vi "Position Removing.vi"(11 "System":string) -> ()   [LabVIEW 2023]
uses:
  <vilib>/Utility/file.llb/Read Delimited Spreadsheet (string).vi
  <vilib>/Utility/file.llb/Write Delimited Spreadsheet (string).vi
panel:
  out "Message":string
  in  "Enter":bool
  in  "Rack Number":i32=1 min=1 max=16 step=1
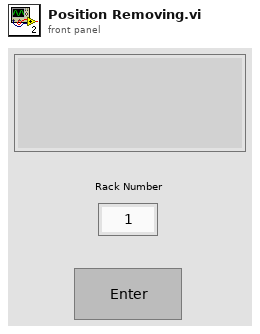
[diagram p1: front panel]
types:
  T1 = enum16{"open", "replace", "create", "open or create", "replace or create", "replace or create with confirmation"}
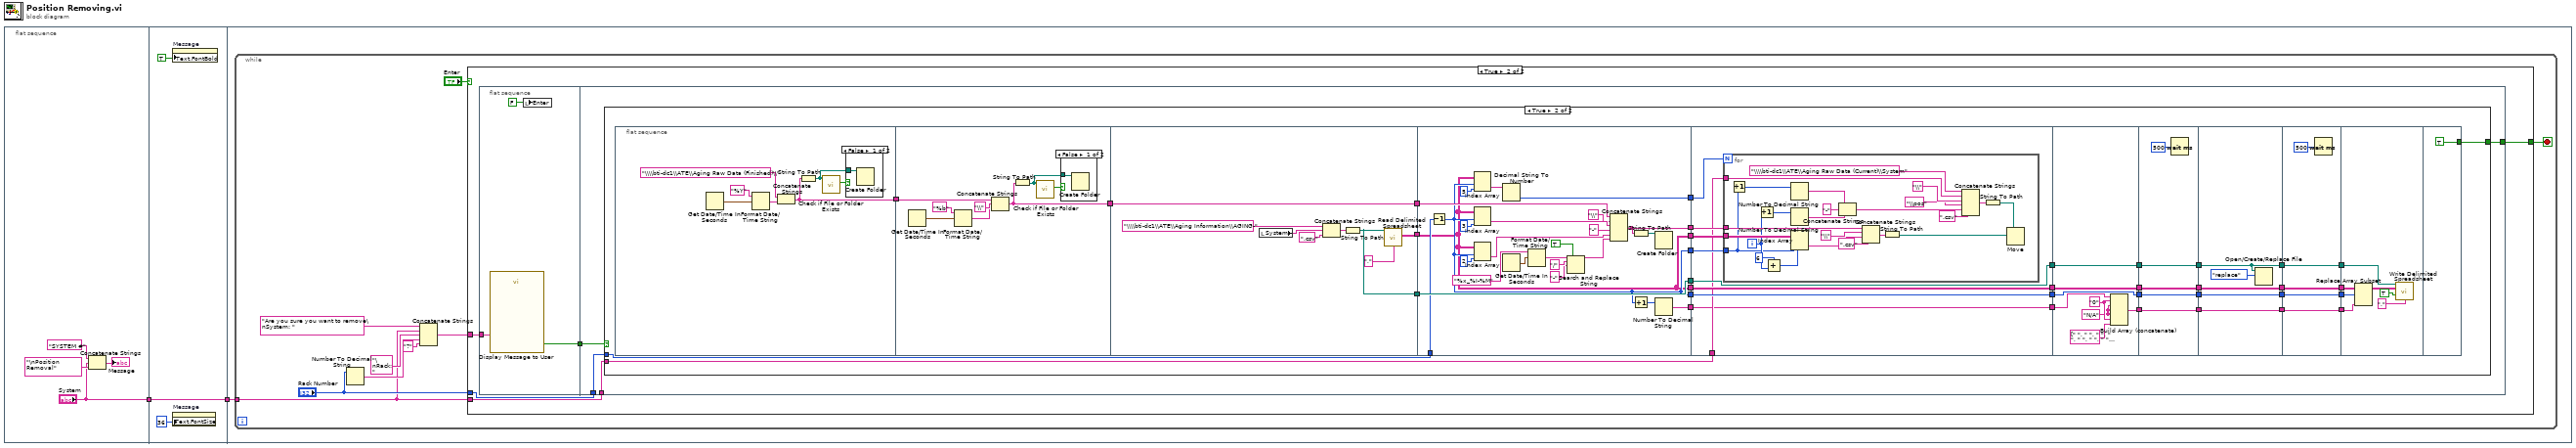
[diagram p0: block diagram]
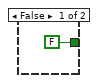
[diagram p2: hidden frame]
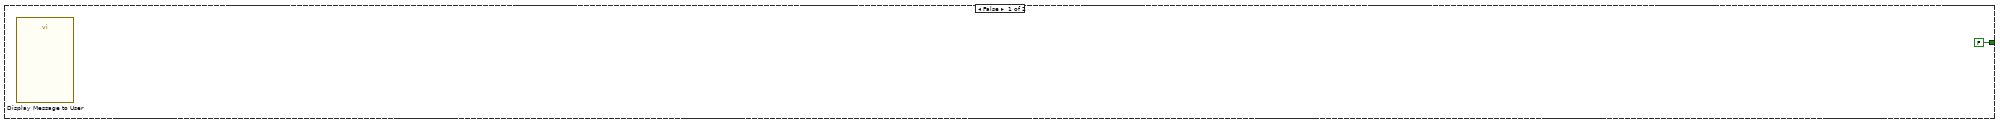
[diagram p3: hidden frame]
diagram:
  n1 = flat-sequence {
    tunnel: ["System"] -> w1
    tunnel: [w7] -> w2
    tunnel: w1 -> [w7]
    tunnel: w2 -> [w10]
    frame #0 {
      n2 = Concatenate Strings("SYSTEM #", "System", "\nPosition Removal") -> (→"Message":string)
    }
    frame #1 {
      n3 = property on="Message" class="Str"("Text.FontBold"=TRUE ("Text.Font:Bold")) -> ()  [unwired: 2 in, 2 out]
      n4 = property on="Message" class="Str"("Text.FontSize"=u32 36 ("Text.Font:Size")) -> ()  [unwired: 2 in, 2 out]
    }
    frame #2 {
      n5 = while {
        tunnel: w10 -> [w11]
        stop <- w18 stop-if-true
        n6 = Number To Decimal String(number="Rack Number") -> (decimal integer string=w16:string)  [unwired: 1 in]
        n7 = Concatenate Strings("Are you sure you want to remove\nSystem: ", w11, "\nRack: ", w16, "?" ("string")) -> (w17:string)
        n8 = case shown="True" "Enter" {
          tunnel: [FALSE w25] -> w18
          tunnel: w17 -> [_ w24]
          tunnel: "Rack Number" -> [_ w22]
          tunnel: w11 -> [_ w21]
          frame False {
          }
          frame True {
            n9 = flat-sequence {
              tunnel: w24 -> [w27]
              tunnel: [w26] -> w23
              tunnel: [w32] -> w25
              tunnel: w23 -> [w31]
              tunnel: w22 -> [w30]
              tunnel: w21 -> [w29]
              frame #0 {
                n10 = call "Display Message to User"("Message"=w27) -> ("Yes"=w26:bool)  [unwired: 9 in, 1 out]
                n11 = local write "Enter"(FALSE ("Enter")) -> ()
              }
              frame #1 {
                n12 = case shown="True" w31 {
                  tunnel: [FALSE w69] -> w32
                  tunnel: w30 -> [_ w48]
                  tunnel: w29 -> [_ w35]
                  frame False {
                    n13 = call "Display Message to User"() -> ()  [unwired: 10 in, 2 out]
                  }
                  frame True {
                    n14 = flat-sequence {
                      tunnel: [w71] -> w52
                      tunnel: w52 -> [w82]
                      tunnel: [w79] -> w51
                      tunnel: [w93] -> w50
                      tunnel: [w92] -> w49
                      tunnel: w51 -> [w87]
                      tunnel: [w87] -> w39
                      tunnel: w50 -> [w97]
                      tunnel: [w97] -> w47
                      tunnel: w49 -> [w119]
                      tunnel: [w119] -> w45
                      tunnel: [w118] -> w43
                      tunnel: [w99] -> w41
                      tunnel: w48 -> [w116]
                      tunnel: w39 -> [w110]
                      tunnel: [w99] -> w38
                      tunnel: [w97] -> w37
                      tunnel: [w101] -> w36
                      tunnel: [w95] -> w34
                      tunnel: w47 -> [w128]
                      tunnel: [w128] -> w46
                      tunnel: w45 -> [w127]
                      tunnel: [w127] -> w44
                      tunnel: w43 -> [w121]
                      tunnel: [w121] -> w42
                      tunnel: w41 -> [w126]
                      tunnel: [w126] -> w40
                      tunnel: w38 -> [w125]
                      tunnel: w37 -> [w124]
                      tunnel: w36 -> [w123]
                      tunnel: w35 -> [w122]
                      tunnel: w34 -> [w120]
                      tunnel: w46 -> [w160]
                      tunnel: [w160] -> w60
                      tunnel: [w153] -> w58
                      tunnel: [w159] -> w56
                      tunnel: w44 -> [w158]
                      tunnel: [w158] -> w54
                      tunnel: w42 -> [w154]
                      tunnel: w40 -> [w153]
                      tunnel: w60 -> [w165]
                      tunnel: [w165] -> w59
                      tunnel: w58 -> [w164]
                      tunnel: [w164] -> w57
                      tunnel: w56 -> [w163]
                      tunnel: [w163] -> w55
                      tunnel: w54 -> [w162]
                      tunnel: [w162] -> w53
                      tunnel: w59 -> [w170]
                      tunnel: [w170] -> w68
                      tunnel: w57 -> [w169]
                      tunnel: [w169] -> w66
                      tunnel: w55 -> [w168]
                      tunnel: [w168] -> w64
                      tunnel: w53 -> [w166]
                      tunnel: [w166] -> w62
                      tunnel: w68 -> [w175]
                      tunnel: [w175] -> w67
                      tunnel: w66 -> [w174]
                      tunnel: [w174] -> w65
                      tunnel: w64 -> [w173]
                      tunnel: [w173] -> w63
                      tunnel: w62 -> [w172]
                      tunnel: [w172] -> w61
                      tunnel: w67 -> [w182]
                      tunnel: w65 -> [w176]
                      tunnel: w63 -> [w181]
                      tunnel: w61 -> [w179]
                      tunnel: [TRUE] -> w69
                      frame #0 {
                        n15 = Get Date/Time In Seconds() -> (seconds since 1Jan1904=w75:timestamp)
                        n16 = Format Date/Time String(time format string (%c)="%Y", seconds (now)=w75) -> (date/time string=w72:string)  [unwired: 1 in]
                        n17 = Concatenate Strings("\\\\bti-dc1\\ATE\\Aging Raw Data (Finished)\\" ("string"), w72) -> (w71:string)
                        n18 = String To Path(string=w71) -> (path=w70:path)
                        n19 = call <vilib>:"Check if File or Folder Exists.vi"("path"=w70) -> ("file or folder exists?"=w76:bool)  [unwired: 8 in, 2 out]
                        n20 = case shown="False" w76 {
                          tunnel: w70 -> [w77 _]
                          frame False {
                            n21 = Create Folder(path (use dialog)=w77) -> ()  [unwired: 2 in, 3 out]
                          }
                          frame True {
                          }
                        }
                      }
                      frame #1 {
                        n22 = Get Date/Time In Seconds() -> (seconds since 1Jan1904=w84:timestamp)
                        n23 = Format Date/Time String(time format string (%c)="%b", seconds (now)=w84) -> (date/time string=w80:string)  [unwired: 1 in]
                        n24 = Concatenate Strings(w82, "\\" ("string"), w80) -> (w79:string)
                        n25 = String To Path(string=w79) -> (path=w78:path)
                        n26 = call <vilib>:"Check if File or Folder Exists.vi"("path"=w78) -> ("file or folder exists?"=w85:bool)  [unwired: 8 in, 2 out]
                        n27 = case shown="False" w85 {
                          tunnel: w78 -> [w86 _]
                          frame False {
                            n28 = Create Folder(path (use dialog)=w86) -> ()  [unwired: 2 in, 3 out]
                          }
                          frame True {
                          }
                        }
                      }
                      frame #2 {
                        n29 = local read "System"() -> (w88:string)
                        n30 = Concatenate Strings("\\\\bti-dc1\\ATE\\Aging Information\\AGING-" ("string"), w88, ".csv" ("string")) -> (w91:string)
                        n31 = String To Path(string=w91) -> (path=w92:path)
                        n32 = call-poly <vilib>:"Read Delimited Spreadsheet.vi"("file path (dialog if empty)"=w92, "delimiter (\\t)"="," ("delimiter (\\t)")) -> ("all rows"=w93:string[][])  [unwired: 8 in, 5 out]
                      }
                      frame #3 {
                        n33 = Decrement(x=w116) -> (x-1=w99:i32)
                        n34 = Index Array(array=w97, index (row)=w99, index (col)=5) -> (element=w96:string)
                        n35 = Index Array(array=w97, index (row)=w99, index (col)=3 ("disabled index (col)")) -> (element=w114:string)
                        n36 = Index Array(array=w97, index (row)=w99, index (col)=2 ("disabled index (col)")) -> (element=w112:string)
                        n37 = Decimal String To Number(string=w96) -> (number=w95:i32)  [unwired: 2 in, 1 out]
                        n38 = Get Date/Time In Seconds() -> (seconds since 1Jan1904=w109:timestamp)
                        n39 = Format Date/Time String(time format string (%c)="%x_%I-%M", seconds (now)=w109) -> (date/time string=w107:string)  [unwired: 1 in]
                        n40 = Search and Replace String(replace all?=TRUE ("replace all? (F)"), input string=w107, search string="/", replace string="-" ("replace string (\"\")")) -> (result string=w103:string)  [unwired: 4 in, 3 out]
                        n41 = Concatenate Strings(w110, "\\" ("string"), w114, "-" ("string"), w112, w103) -> (w101:string)
                        n42 = String To Path(string=w101) -> (path=w102:path)
                        n43 = Increment(x=w99) -> (x+1=w100:i32)
                        n44 = Create Folder(path (use dialog)=w102) -> ()  [unwired: 2 in, 3 out]
                        n45 = Number To Decimal String(number=w100) -> (decimal integer string=w118:string)  [unwired: 1 in]
                      }
                      frame #4 {
                        n46 = for {
                          N: w120 -> [_]
                          tunnel: w125 -> [w135]
                          tunnel: w124 -> [w150]
                          tunnel: w123 -> [w149]
                          tunnel: w122 -> [w145]
                          i -> [w142]
                          n47 = Increment(x=w135) -> (x+1=w134:i32)
                          n48 = Increment(x=w142) -> (x+1=w137:i32)
                          n49 = Add(x=6, y=w142) -> (x+y=w151:i32)
                          n50 = Number To Decimal String(number=w134) -> (decimal integer string=w133:string)  [unwired: 1 in]
                          n51 = Number To Decimal String(number=w137) -> (decimal integer string=w143:string)  [unwired: 1 in]
                          n52 = Index Array(array=w150, index (row)=w135, index (col)=w151) -> (element=w147:string)
                          n53 = Concatenate Strings(w133, "-" ("string"), w143) -> (w132:string)
                          n54 = Concatenate Strings(w149, "\\" ("string"), w147, ".csv" ("string")) -> (w130:string)
                          n55 = String To Path(string=w130) -> (path=w129:path)
                          n56 = Concatenate Strings("\\\\bti-dc1\\ATE\\Aging Raw Data (Current)\\System", w145, "\\" ("string"), "\\pos" ("string"), w132, ".csv" ("string")) -> (w141:string)
                          n57 = String To Path(string=w141) -> (path=w138:path)
                          n58 = Move(source path=w138, 10:w129) -> ()  [unwired: 3 in, 3 out]
                        }
                      }
                      frame #5 {
                        w155 = "N/A" ("element")
                        w156 = "0" ("element")
                        n59 = Build Array (concatenate)(w154, w156, w155, w155, w155, w156, string[] [" ", " ", " ", " ", " ", " ", " ", " ", " ", " ", " ", "", "", "", "", "", "", "", "", "", "", "", "", "", "", "", "", "", "", "", "", "", "", "", "", "", "", "", "", "", " "] ("array")) -> (w159:string[])
                      }
                      frame #6 {
                        n60 = Wait (ms)(milliseconds to wait=u32 500) -> ()  [unwired: 1 out]
                      }
                      frame #7 {
                        n61 = Open/Create/Replace File(file path (use dialog)=w166, operation (0:open)=T1."replace") -> ()  [unwired: 4 in, 3 out]
                      }
                      frame #8 {
                        n62 = Wait (ms)(milliseconds to wait=u32 500) -> ()  [unwired: 1 out]
                      }
                      frame #9 {
                        n63 = Replace Array Subset(array=w182, new element=w181, index (row)=w176) -> (w180:string[][])  [unwired: 1 in]
                        n64 = call-poly <vilib>:"Write Delimited Spreadsheet.vi"("file path (dialog if empty)"=w179, "2D data"=w180, "append to file? (new file:F)"=TRUE, "delimiter (\\t)"="," ("delimiter (\\t)")) -> ()  [unwired: 10 in, 2 out]
                      }
                      frame #10 {
                      }
                    }
                  }
                }
              }
            }
          }
        }
      }
    }
  }
